vi "废液监测界面.vi"() -> ()   [LabVIEW 2016, in "环境动力监测库.lvlib"]
panel:
  out "x+1":u32
  in  "解除告警":bool
  out "告警内容":string
  out "废液监测":bool caption="状态"
  # "废液监测"
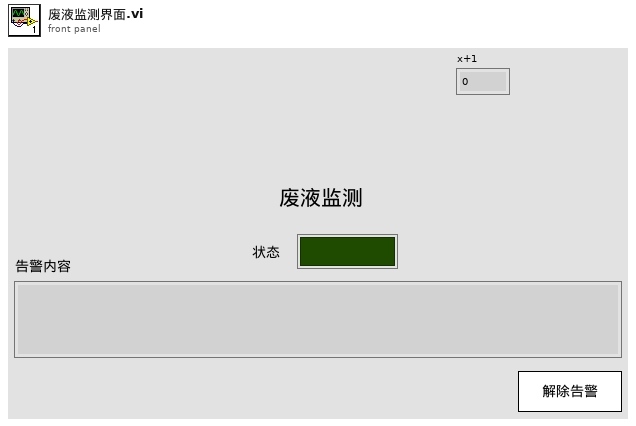
[diagram p1: front panel]
types:
  T1 = cluster{"漏水监测配置":cluster{"监测项描述:输出":string, "端口:":enum16{"AI0", "AI1", "AI2", "AI3", "AI4", "DI0", "DI1", "DI2", "DI3", "DI4", "DI5", "DI6", "DI7", "DO0", "DO1", "DO2", "DO3", "DO4", "DO5", "DO6", "DO7", "X0", "X1", "X2", "X3", "X4", "X5", "X6", "X7", "X8", "X9", "X10", "X11", "X12", "X13", "X14", "X15", "X16", "X17", "X18", "X19", "X20", "X21", "X22", "X23"}, "告警参数:":enum32{"禁用告警", "闭合告警", "断开告警"}, "传感器型号:":enum16{"PLC", "ZLAN", "ART"}, "声光告警启用":bool}, "门禁开关监测配置":cluster{"监测项描述:输出":string, "端口:":enum16{"AI0", "AI1", "AI2", "AI3", "AI4", "DI0", "DI1", "DI2", "DI3", "DI4", "DI5", "DI6", "DI7", "DO0", "DO1", "DO2", "DO3", "DO4", "DO5", "DO6", "DO7", "X0", "X1", "X2", "X3", "X4", "X5", "X6", "X7", "X8", "X9", "X10", "X11", "X12", "X13", "X14", "X15", "X16", "X17", "X18", "X19", "X20", "X21", "X22", "X23"}, "告警参数:":enum32{"禁用告警", "闭合告警", "断开告警"}, "传感器型号:":enum16{"PLC", "ZLAN", "ART"}, "声光告警启用":bool}, "门禁开关监测配置2":cluster{"监测项描述:输出":string, "端口:":enum16{"AI0", "AI1", "AI2", "AI3", "AI4", "DI0", "DI1", "DI2", "DI3", "DI4", "DI5", "DI6", "DI7", "DO0", "DO1", "DO2", "DO3", "DO4", "DO5", "DO6", "DO7", "X0", "X1", "X2", "X3", "X4", "X5", "X6", "X7", "X8", "X9", "X10", "X11", "X12", "X13", "X14", "X15", "X16", "X17", "X18", "X19", "X20", "X21", "X22", "X23"}, "告警参数:":enum32{"禁用告警", "闭合告警", "断开告警"}, "传感器型号:":enum16{"PLC", "ZLAN", "ART"}, "声光告警启用":bool}, "温湿度监测配置":cluster{"监测项描述:输出":string, "端口:":enum16{"AI0", "AI1", "AI2", "AI3", "AI4", "DI0", "DI1", "DI2", "DI3", "DI4", "DI5", "DI6", "DI7", "DO0", "DO1", "DO2", "DO3", "DO4", "DO5", "DO6", "DO7", "X0", "X1", "X2", "X3", "X4", "X5", "X6", "X7", "X8", "X9", "X10", "X11", "X12", "X13", "X14", "X15", "X16", "X17", "X18", "X19", "X20", "X21", "X22", "X23"}, "告警参数:":enum32{"禁用告警", "闭合告警", "断开告警"}, "传感器型号:":enum16{"PLC", "ZLAN", "ART"}, "声光告警启用":bool}, "烟雾监测配置":cluster{"监测项描述:输出":string, "端口:":enum16{"AI0", "AI1", "AI2", "AI3", "AI4", "DI0", "DI1", "DI2", "DI3", "DI4", "DI5", "DI6", "DI7", "DO0", "DO1", "DO2", "DO3", "DO4", "DO5", "DO6", "DO7", "X0", "X1", "X2", "X3", "X4", "X5", "X6", "X7", "X8", "X9", "X10", "X11", "X12", "X13", "X14", "X15", "X16", "X17", "X18", "X19", "X20", "X21", "X22", "X23"}, "告警参数:":enum32{"禁用告警", "闭合告警", "断开告警"}, "传感器型号:":enum16{"PLC", "ZLAN", "ART"}, "声光告警启用":bool}, "冰箱监测配置":cluster{"监测项描述:输出":string, "端口:":enum16{"AI0", "AI1", "AI2", "AI3", "AI4", "DI0", "DI1", "DI2", "DI3", "DI4", "DI5", "DI6", "DI7", "DO0", "DO1", "DO2", "DO3", "DO4", "DO5", "DO6", "DO7", "X0", "X1", "X2", "X3", "X4", "X5", "X6", "X7", "X8", "X9", "X10", "X11", "X12", "X13", "X14", "X15", "X16", "X17", "X18", "X19", "X20", "X21", "X22", "X23"}, "告警参数:":enum32{"禁用告警", "闭合告警", "断开告警"}, "传感器型号:":enum16{"PLC", "ZLAN", "ART"}, "声光告警启用":bool}, "排气扇监测配置":cluster{"监测项描述:输出":string, "端口:":enum16{"AI0", "AI1", "AI2", "AI3", "AI4", "DI0", "DI1", "DI2", "DI3", "DI4", "DI5", "DI6", "DI7", "DO0", "DO1", "DO2", "DO3", "DO4", "DO5", "DO6", "DO7", "X0", "X1", "X2", "X3", "X4", "X5", "X6", "X7", "X8", "X9", "X10", "X11", "X12", "X13", "X14", "X15", "X16", "X17", "X18", "X19", "X20", "X21", "X22", "X23"}, "告警参数:":enum32{"禁用告警", "闭合告警", "断开告警"}, "传感器型号:":enum16{"PLC", "ZLAN", "ART"}, "声光告警启用":bool}, "红外入侵监测配置":cluster{"监测项描述:输出":string, "端口:":enum16{"AI0", "AI1", "AI2", "AI3", "AI4", "DI0", "DI1", "DI2", "DI3", "DI4", "DI5", "DI6", "DI7", "DO0", "DO1", "DO2", "DO3", "DO4", "DO5", "DO6", "DO7", "X0", "X1", "X2", "X3", "X4", "X5", "X6", "X7", "X8", "X9", "X10", "X11", "X12", "X13", "X14", "X15", "X16", "X17", "X18", "X19", "X20", "X21", "X22", "X23"}, "告警参数:":enum32{"禁用告警", "闭合告警", "断开告警"}, "传感器型号:":enum16{"PLC", "ZLAN", "ART"}, "声光告警启用":bool}, "振动监测配置":cluster{"监测项描述:输出":string, "端口:":enum16{"AI0", "AI1", "AI2", "AI3", "AI4", "DI0", "DI1", "DI2", "DI3", "DI4", "DI5", "DI6", "DI7", "DO0", "DO1", "DO2", "DO3", "DO4", "DO5", "DO6", "DO7", "X0", "X1", "X2", "X3", "X4", "X5", "X6", "X7", "X8", "X9", "X10", "X11", "X12", "X13", "X14", "X15", "X16", "X17", "X18", "X19", "X20", "X21", "X22", "X23"}, "告警参数:":enum32{"禁用告警", "闭合告警", "断开告警"}, "传感器型号:":enum16{"PLC", "ZLAN", "ART"}, "声光告警启用":bool}, "废液监测配置":cluster{"监测项描述:输出":string, "端口:":enum16{"AI0", "AI1", "AI2", "AI3", "AI4", "DI0", "DI1", "DI2", "DI3", "DI4", "DI5", "DI6", "DI7", "DO0", "DO1", "DO2", "DO3", "DO4", "DO5", "DO6", "DO7", "X0", "X1", "X2", "X3", "X4", "X5", "X6", "X7", "X8", "X9", "X10", "X11", "X12", "X13", "X14", "X15", "X16", "X17", "X18", "X19", "X20", "X21", "X22", "X23"}, "告警参数:":enum32{"禁用告警", "闭合告警", "断开告警"}, "传感器型号:":enum16{"PLC", "ZLAN", "ART"}, "声光告警启用":bool}, "废液监测配置2":cluster{"监测项描述:输出":string, "端口:":enum16{"AI0", "AI1", "AI2", "AI3", "AI4", "DI0", "DI1", "DI2", "DI3", "DI4", "DI5", "DI6", "DI7", "DO0", "DO1", "DO2", "DO3", "DO4", "DO5", "DO6", "DO7", "X0", "X1", "X2", "X3", "X4", "X5", "X6", "X7", "X8", "X9", "X10", "X11", "X12", "X13", "X14", "X15", "X16", "X17", "X18", "X19", "X20", "X21", "X22", "X23"}, "告警参数:":enum32{"禁用告警", "闭合告警", "断开告警"}, "传感器型号:":enum16{"PLC", "ZLAN", "ART"}, "声光告警启用":bool}}
  T2 = cluster{"监测项描述:输出":string, "端口:":enum16{"AI0", "AI1", "AI2", "AI3", "AI4", "DI0", "DI1", "DI2", "DI3", "DI4", "DI5", "DI6", "DI7", "DO0", "DO1", "DO2", "DO3", "DO4", "DO5", "DO6", "DO7", "X0", "X1", "X2", "X3", "X4", "X5", "X6", "X7", "X8", "X9", "X10", "X11", "X12", "X13", "X14", "X15", "X16", "X17", "X18", "X19", "X20", "X21", "X22", "X23"}, "告警参数:":enum32{"禁用告警", "闭合告警", "断开告警"}, "传感器型号:":enum16{"PLC", "ZLAN", "ART"}, "声光告警启用":bool}
  T3 = enum16{"AI0", "AI1", "AI2", "AI3", "AI4", "DI0", "DI1", "DI2", "DI3", "DI4", "DI5", "DI6", "DI7", "DO0", "DO1", "DO2", "DO3", "DO4", "DO5", "DO6", "DO7", "X0", "X1", "X2", "X3", "X4", "X5", "X6", "X7", "X8", "X9", "X10", "X11", "X12", "X13", "X14", "X15", "X16", "X17", "X18", "X19", "X20", "X21", "X22", "X23"}
  T4 = cluster{"漏水监测输出":cluster{"漏水监测告警":bool, "告警内容":string}, "门禁监测输出":cluster{"门禁监测告警":bool, "告警内容":string}, "门禁监测输出2":cluster{"门禁监测告警":bool, "告警内容":string}, "温湿度监测输出":cluster{"温湿度监测告警":bool, "告警内容":string}, "烟雾监测输出":cluster{"烟雾监测告警":bool, "告警内容":string}, "空调监测输出":cluster{"空调监测告警":bool, "告警内容":string}, "自动重合闸输出":cluster{"自动重合闸告警":bool, "告警内容":string}, "红外入侵输出":cluster{"红外入侵告警":bool, "告警内容":string}, "振动输出":cluster{"振动告警":bool, "告警内容":string}, "UPS输出":cluster{"UPS告警":bool, "告警内容":string}, "蓄电池输出":cluster{"蓄电池告警":bool, "告警内容":string}, "蓄电池输出2":cluster{"蓄电池告警":bool, "告警内容":string}, "GPS输出":cluster{"定位告警":bool, "告警内容":string}, "北斗输出":cluster{"定位告警":bool, "告警内容":string}, "气象输出":cluster{"气象告警":bool, "告警内容":string}, "废液输出":cluster{"废液告警":bool, "告警内容":string}, "废液输出2":cluster{"废液告警":bool, "告警内容":string}}
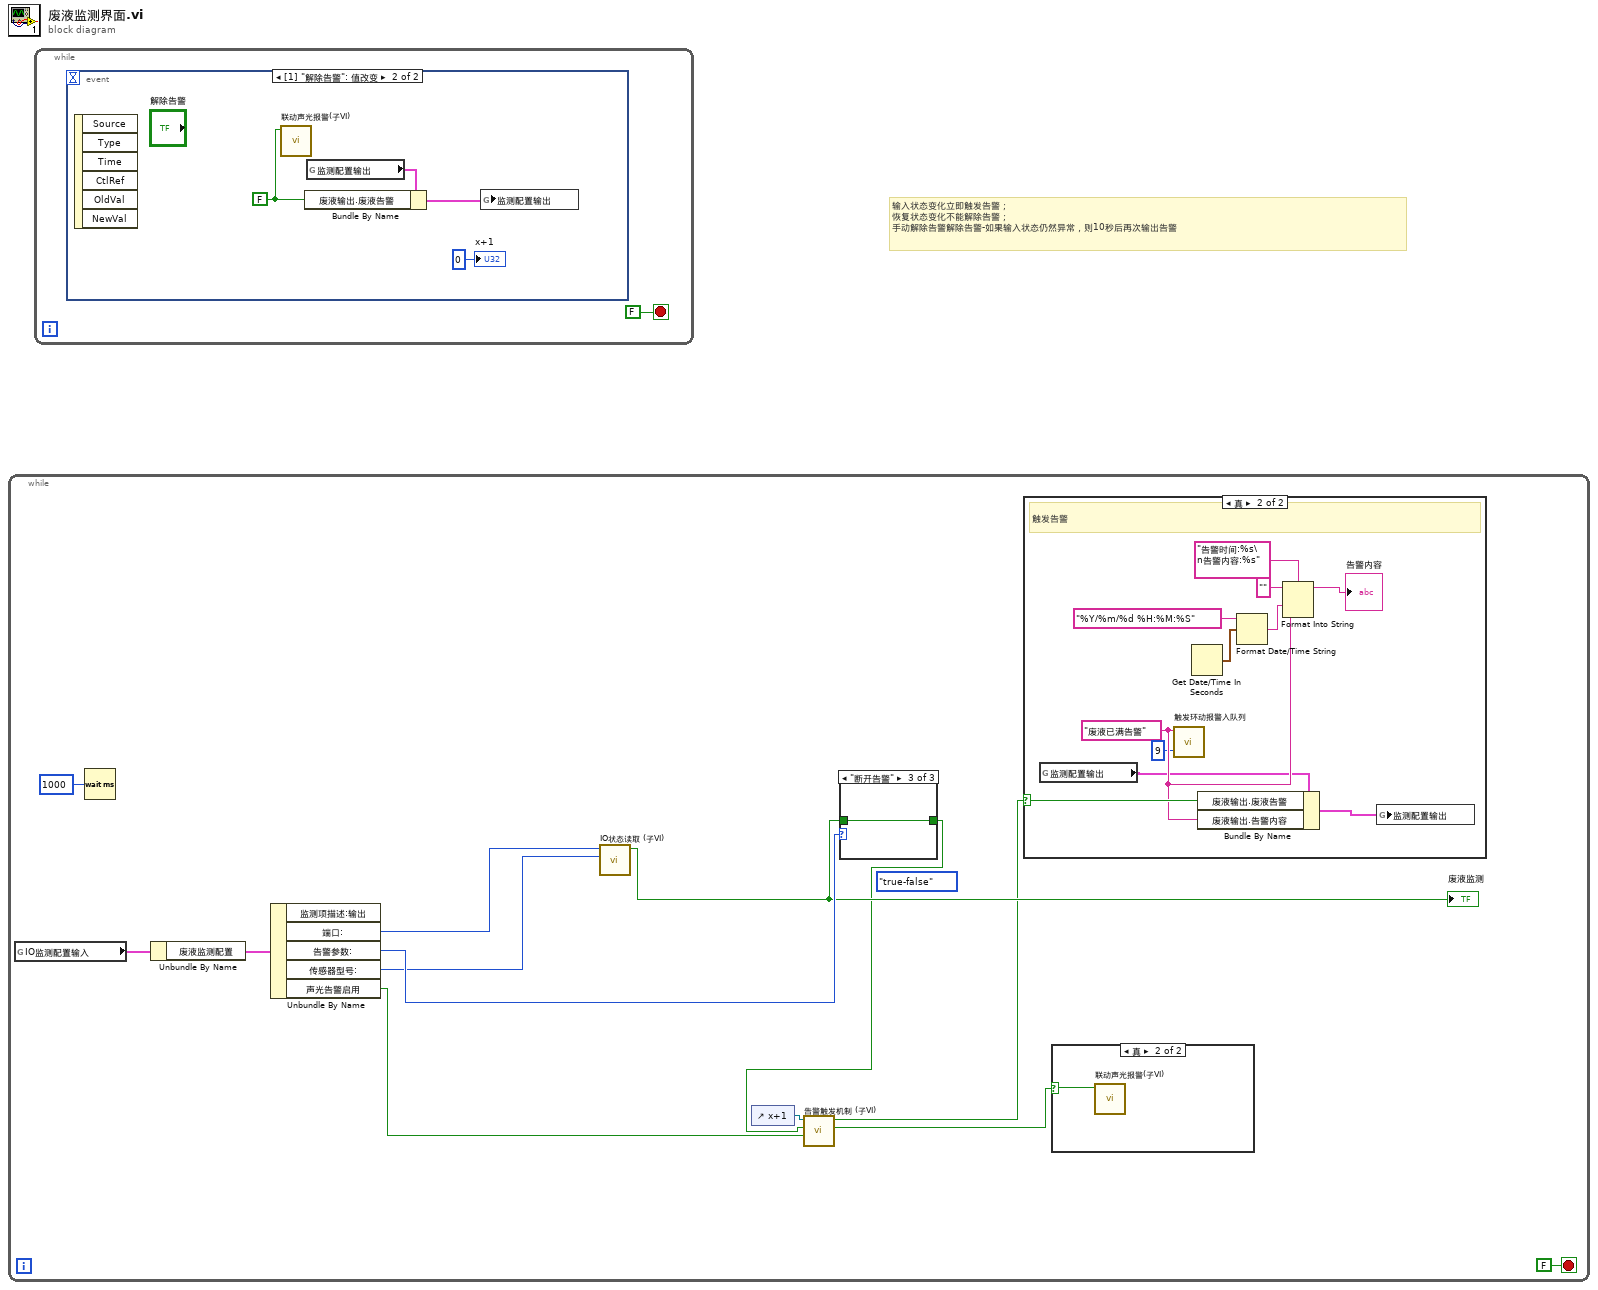
[diagram p0: block diagram]
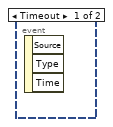
[diagram p2: hidden frame]
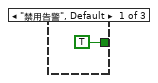
[diagram p5: hidden frame]
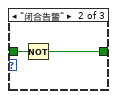
[diagram p6: hidden frame]
diagram:
  # "输入状态变化立即触发告警；\n恢复状态变化不能解除告警；\n手动解除告警解除告警-如果输入状态仍然异常，则10秒后再次输出告警"
  n1 = while {
    stop <- FALSE stop-if-true
    (unwired) enum16{"either", "false-true", "true-false"}."true-false" ("direction")
    n2 = global read "断电保存全局变量.vi" "IO监测配置输入"() -> (w6:T1)
    n3 = Wait (ms)(milliseconds to wait=u32 1000 ("等待时间（毫秒）")) -> ()  [unwired: 1 out]
    n4 = Unbundle By Name(w6) -> ("废液监测配置"=w13:T2)
    n5 = Unbundle By Name(w13) -> ("端口:"=w9:T3, "告警参数:"=w12:enum32{"禁用告警", "闭合告警", "断开告警"}, "传感器型号:"=w8:enum16{"PLC", "ZLAN", "ART"}, "声光告警启用"=w5:bool)  [unwired: 1 out]
    n6 = call "IO状态读取 (子VI).vi"("传感器型号:"=w8, "端口:"=w9) -> ("布尔"=w7:bool)  [unwired: 9 in]
    "废液监测" <- w7
    n7 = control-ref of="x+1"() -> (w1:refnum<vi>)
    n8 = case shown="\"断开告警\"" w12 {
      tunnel: w7 -> [_ w28 w29]
      tunnel: [TRUE ("漏水监测输出") w27 w29] -> w2
      frame "禁用告警", Default {
      }
      frame "闭合告警" {
        n9 = Not(x=w28) -> (.not. x?=w27:bool)
      }
      frame "断开告警" {
      }
    }
    n10 = call "告警触发机制 (子VI).vi"("声光告警启用"=w5, "状态输出"=w2, "Digital输入"=w1) -> ("声光告警"=w4:bool, "触发告警"=w3:bool)  [unwired: 7 in]
    n11 = case shown="真" w3 {
      selector: w3 -> [_ w25]
      frame False {
      }
      frame True {
        w19 = "废液已满告警" ("报警内容")
        # "触发告警"
        n12 = global read "内部交互全局变量.vi" "监测配置输出"() -> (w16:T4)
        n13 = call "触发环动报警入队列.vi"("code"=9, "报警内容"=w19) -> ()  [unwired: 10 in]
        n14 = Get Date/Time In Seconds() -> (seconds since 1Jan1904=w22:timestamp)
        n15 = Bundle By Name(cluster=w16, "废液输出.废液告警"=w25, "废液输出.告警内容"=w19) -> (w17:T4)
        n16 = Format Date/Time String(time format string (%c)="%Y/%m/%d %H:%M:%S" ("时间格式字符串(%c)"), seconds (now)=w22) -> (date/time string=w24:string)  [unwired: 1 in]
        n17 = Format Into String(format string="告警时间:%s\n告警内容:%s" ("格式字符串"), initial string="" ("初始字符串"), w24, w19) -> (resulting string=→"告警内容":string)  [unwired: 1 in, 1 out]
        n18 = global write "内部交互全局变量.vi" "监测配置输出"(w17) -> ()
      }
    }
    n19 = case shown="真" w4 {
      selector: w4 -> [_ w14]
      frame False {
      }
      frame True {
        n20 = call "联动声光报警(子VI).vi"("布尔"=w14) -> ()  [unwired: 11 in]
      }
    }
  }
  n21 = while {
    stop <- FALSE stop-if-true
    n22 = event shown="[1] \"解除告警\": 值改变" {
      selector: _ -> [_ _]
      dyn-events: _ -> [_ _]
      timeout: _ -> [_ _]
      event Timeout {
        n23 = event-data() -> ()  [unwired: 1 in, 3 out]
      }
      event "解除告警": Value Change {
        w34 = FALSE
        n24 = event-data() -> ()  [unwired: 1 in, 6 out]
        n25 = call "联动声光报警(子VI).vi"("布尔"=w34) -> ()  [unwired: 11 in]
        n26 = global read "内部交互全局变量.vi" "监测配置输出"() -> (w32:T4)
        n27 = Bundle By Name(cluster=w32, "废液输出.废液告警"=w34) -> (w31:T4)
        n28 = global write "内部交互全局变量.vi" "监测配置输出"(w31) -> ()
        "x+1" <- u32 0 ("x+1")
      }
    }
  }
